vi "ReturnUniqueChild.vi"(11 "Array In":string[][](array[string])) -> (2 "Unique Child":string[][](array[string]), 3 "Array Out":string[][](array[string]))   [LabVIEW 2020, in "Mermaid.lvlib" / "Application.lvclass"]
uses:
  Application.lvclass
  Application.lvclass/Application.ctl
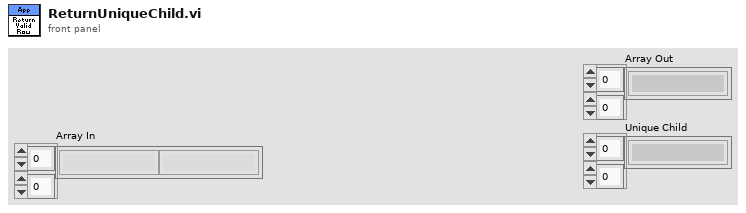
[diagram p1: front panel]
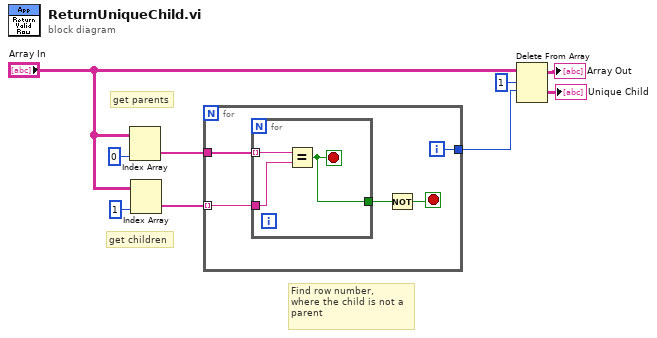
[diagram p0: block diagram]
diagram:
  # "Find row number,\nwhere the child is not a\nparent"
  # "get children"
  # "get parents"
  n1 = Index Array(array="Array In", index (col)=0 ("disabled index (col)")) -> (element=w6:string[])  [unwired: 1 in]
  n2 = Index Array(array="Array In", index (col)=1 ("disabled index (col)")) -> (element=w7:string[])  [unwired: 1 in]
  n3 = for {
    tunnel: w7 -> [w13] mode=indexing
    tunnel: w6 -> [w14]
    tunnel: [w10] -> w4
    i -> [w10]
    stop <- w11 stop-if-true
    n4 = for {
      tunnel: w14 -> [w17] mode=indexing
      tunnel: w13 -> [w16]
      tunnel: [w15] -> w12
      stop <- w15 stop-if-true
      n5 = Equal?(x=w17, y=w16) -> (x = y?=w15:bool)
    }
    n6 = Not(x=w12) -> (.not. x?=w11:bool)
  }
  n7 = Delete From Array(array="Array In", length=1, index (row)=w4) -> (deleted portion=→"Unique Child":string[][], array with subset deleted=→"Array Out":string[][])  [unwired: 1 in]
